vi "Is Cooler On.vi"(8 "error in (no error)":errorcluster, 11 "iCoolerStatus":i32) -> (0 "error out":errorcluster, 2 "function return":u32, 3 "iCoolerStatus out":i32)   [LabVIEW 2014, in "atmcd32d.lvlib"]
doc: "unsigned int WINAPI IsCoolerOn(int * iCoolerStatus);"
uses:
  atmcd32d.lvlib
  atmcd32d.dll
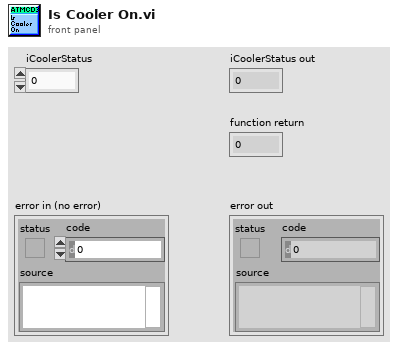
[diagram p1: front panel]
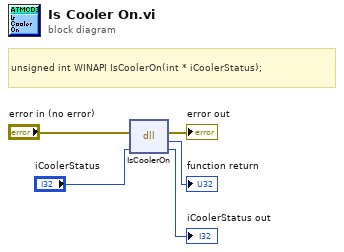
[diagram p0: block diagram]
diagram:
  # "unsigned int WINAPI IsCoolerOn(int * iCoolerStatus);"
  n1 = dll-call lib="C:/Users/Bakir/Documents/Lambda2-Testing/lib/Andorlib/atmcd32d.*" fn="IsCoolerOn"(error in="error in (no error)", "iCoolerStatus"="iCoolerStatus") -> (error out=→"error out":errorcluster, →"function return":u32, "iCoolerStatus"=→"iCoolerStatus out":i32)  [unwired: 2 in, 1 out]
